vi "Init.vi"(8 "Error In":errorcluster, 10 "IConfigure":refnum<class "IConfigure.lvclass">, 11 "Object in":refnum<class "PXIe-5172 Simulated.lvclass">) -> (0 "Error Out":errorcluster, 3 "Object out":refnum<class "PXIe-5172 Simulated.lvclass">)   [LabVIEW 2023, in "PXIe-5172 Simulated.lvlib" / "PXIe-5172 Simulated.lvclass"]
uses:
  PXIe-5172 Simulated.lvclass
  Scope PXI/Scope PXI.lvclass
  D:/git/HAL/Scope PXI/Scope PXI.lvclass
  D:/git/HAL/Scope Base/Scope Base.lvclass
  D:/git/HAL/Instrument/Instrument.lvclass
  D:/git/HAL/Interfaces/IRead Voltage/IRead Voltage.lvclass
  D:/git/HAL/Interfaces/IScope/IScope.lvclass
  D:/git/HAL/Devices/PXIe-5172 Simulated/PXIe-5172 Simulated.lvclass
  Interfaces/IConfigure/IConfigure.lvclass
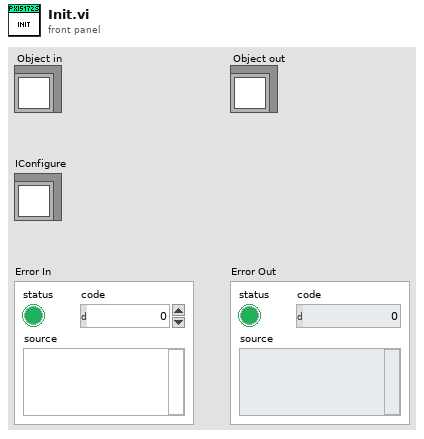
[diagram p1: front panel]
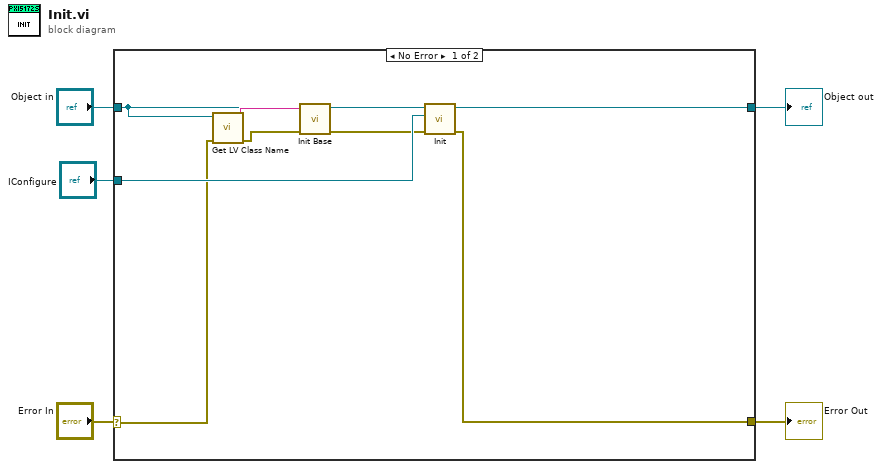
[diagram p0: block diagram]
diagram:
  n1 = case shown="No Error" "Error In" {
    selector: "Error In" -> [w8 w15]
    tunnel: [w10 w16] -> w5
    tunnel: "Object in" -> [w6 w16]
    tunnel: [w11 w15] -> w2
    tunnel: "IConfigure" -> [w13 _]
    frame No Error {
      n2 = call <vilib>:"Get LV Class Name.vi"("error in (no error)"=w8, "object"=w6) -> ("error out"=w7:errorcluster, "class name"=w9:string)  [unwired: 8 in]
      n3 = call-dynamic "Init Base.vi"("Error In"=w7, 10:w9, "object in"=w6) -> ("Error Out"=w12:errorcluster, "object out"=w14:refnum<class "PXIe-5172 Simulated.lvclass">)  [unwired: 7 in]
      n4 = call-parent "Init.vi"("Error In"=w12, "IConfigure"=w13, "object in"=w14) -> ("Error Out"=w11:errorcluster, "object out"=w10:refnum<class "PXIe-5172 Simulated.lvclass">)  [unwired: 7 in]
    }
    frame Error {
    }
  }
  "Object out" <- w5
  "Error Out" <- w2
